vi "labview_python_send_serial_hex.vi"() -> ()   [LabVIEW 2025]
panel:
  in  "H2 Order":dbl
  in  "H2 Phase":dbl
  in  "H2 Volt":dbl
  in  "H1 Order":dbl
  in  "H1 Phase":dbl
  in  "H1 Volt":dbl
  in  "Freq Dev":dbl
  in  "Mod Freq":dbl
  in  "Mod Amp":dbl
  in  "ROCOF rate":dbl
  in  "Time":dbl
  in  "Frequency Step":dbl
  in  "Phase Step":dbl
  in  "Voltage Step":dbl
  in  "Test Type":u16(ring) items=["Steady State", "Voltage Step", "Phase Step", "Frequency Step", "Frequency Ramp", "Amplitude Modulation", "Phase Modulation", "Harmonics"]
  in  "Phase":dbl=90.0
  in  "Frequency":dbl=50.0
  in  "Voltage":dbl=1.0
  out "Debug":string
  in  "Python Version":T1(ring)=enum."3.12"
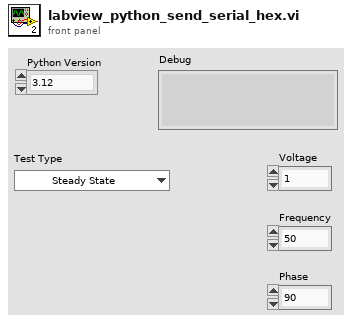
[diagram p1: front panel]
types:
  T1 = enum16{"3.6", "3.7", "3.8", "3.9", "3.10", "3.11", "3.12"}
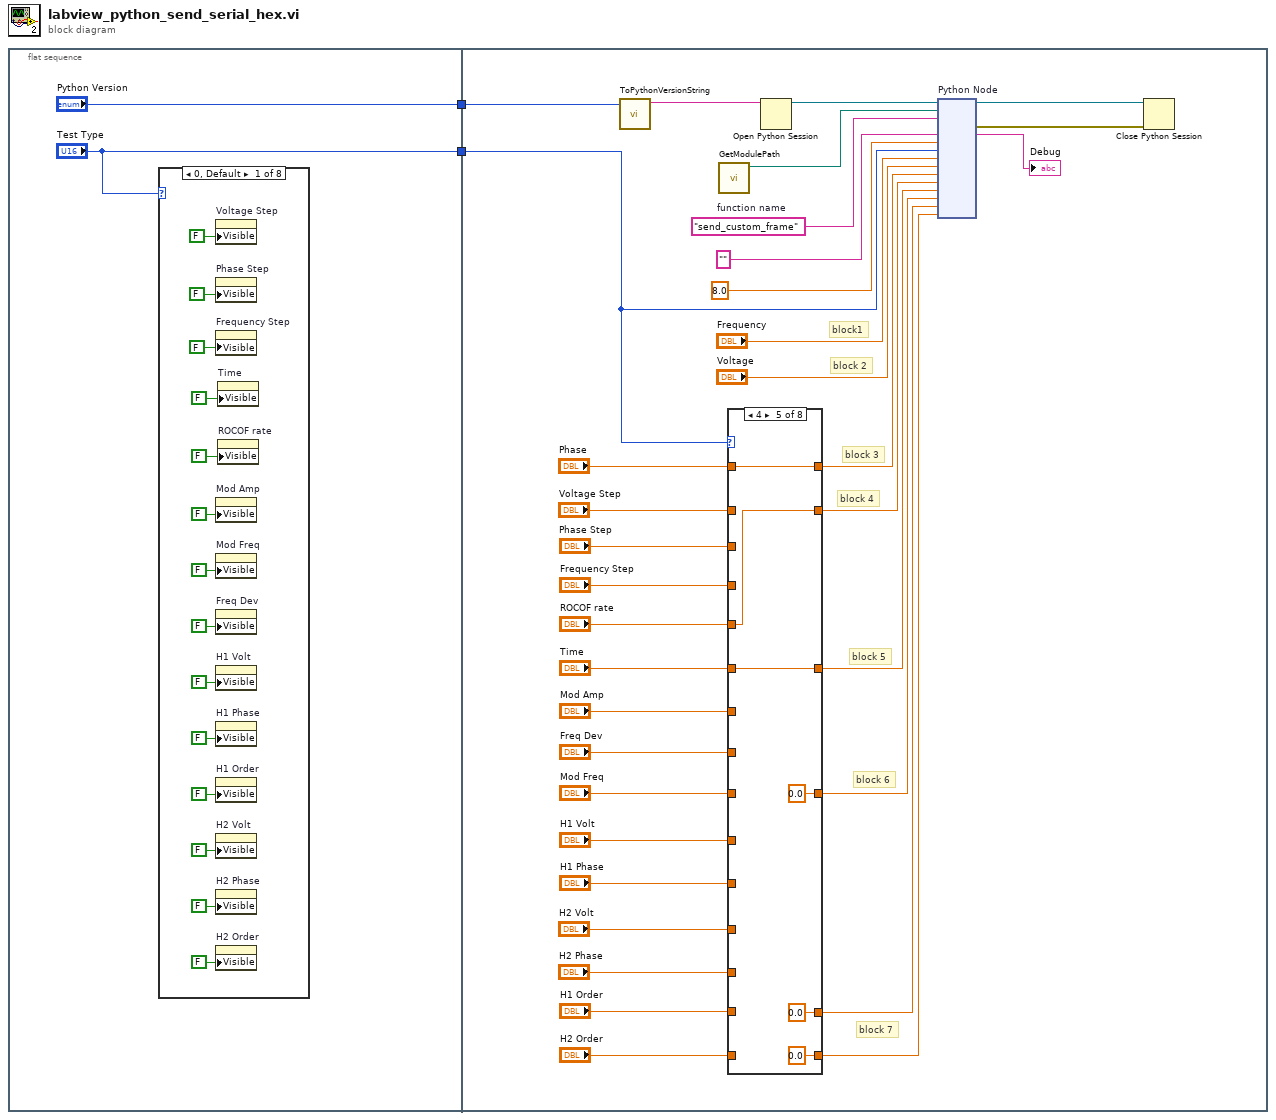
[diagram p0: block diagram]
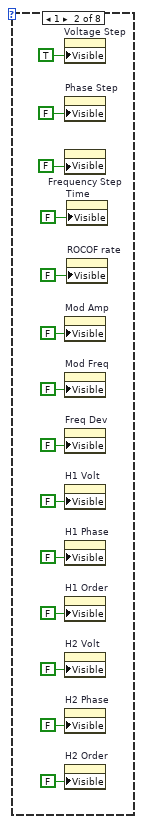
[diagram p2: hidden frame]
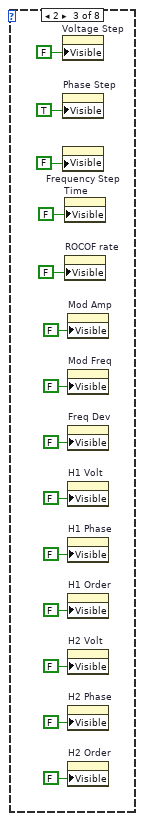
[diagram p3: hidden frame]
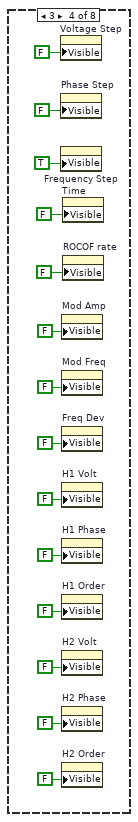
[diagram p4: hidden frame]
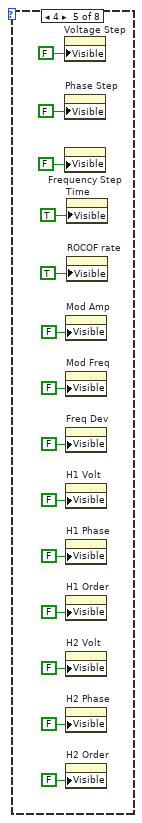
[diagram p5: hidden frame]
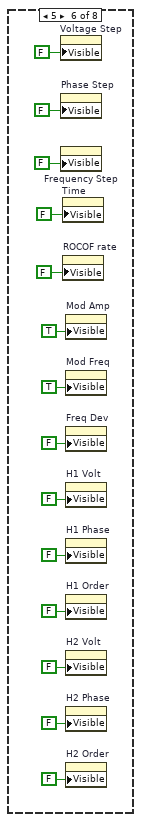
[diagram p6: hidden frame]
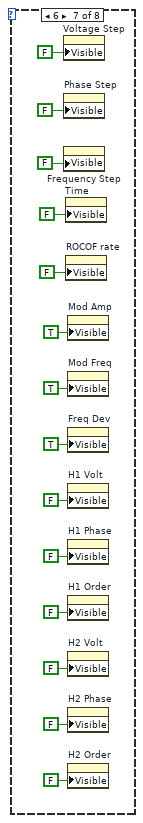
[diagram p7: hidden frame]
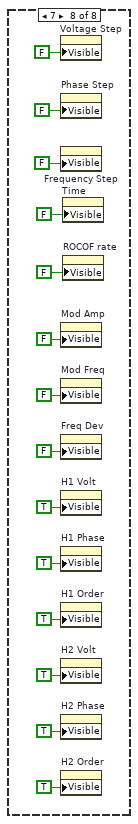
[diagram p8: hidden frame]
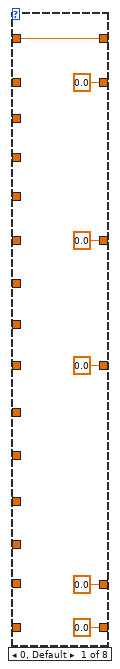
[diagram p9: hidden frame]
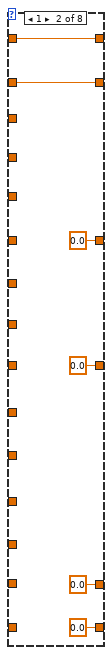
[diagram p10: hidden frame]
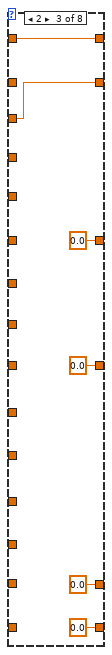
[diagram p11: hidden frame]
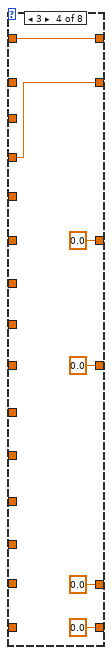
[diagram p12: hidden frame]
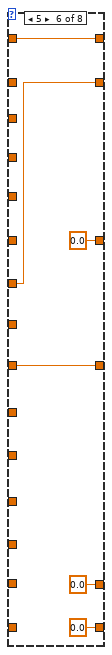
[diagram p13: hidden frame]
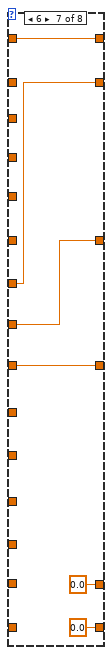
[diagram p14: hidden frame]
diagram:
  n1 = flat-sequence {
    tunnel: ["Python Version"] -> w2
    tunnel: ["Test Type"] -> w1
    tunnel: w2 -> [w142]
    tunnel: w1 -> [w138]
    frame #0 {
      n2 = case shown="0, Default" "Test Type" {
        frame 0, Default {
          n3 = property on="Voltage Step" class="DigNum (strict)"("Visible"=FALSE) -> ()  [unwired: 2 in, 2 out]
          n4 = property on="Phase Step" class="DigNum (strict)"("Visible"=FALSE) -> ()  [unwired: 2 in, 2 out]
          n5 = property on="Frequency Step" class="DigNum (strict)"("Visible"=FALSE) -> ()  [unwired: 2 in, 2 out]
          n6 = property on="Mod Amp" class="DigNum (strict)"("Visible"=FALSE) -> ()  [unwired: 2 in, 2 out]
          n7 = property on="Mod Freq" class="DigNum (strict)"("Visible"=FALSE) -> ()  [unwired: 2 in, 2 out]
          n8 = property on="Freq Dev" class="DigNum (strict)"("Visible"=FALSE) -> ()  [unwired: 2 in, 2 out]
          n9 = property on="H1 Volt" class="DigNum (strict)"("Visible"=FALSE) -> ()  [unwired: 2 in, 2 out]
          n10 = property on="H1 Phase" class="DigNum (strict)"("Visible"=FALSE) -> ()  [unwired: 2 in, 2 out]
          n11 = property on="H1 Order" class="DigNum (strict)"("Visible"=FALSE) -> ()  [unwired: 2 in, 2 out]
          n12 = property on="H2 Volt" class="DigNum (strict)"("Visible"=FALSE) -> ()  [unwired: 2 in, 2 out]
          n13 = property on="H2 Phase" class="DigNum (strict)"("Visible"=FALSE) -> ()  [unwired: 2 in, 2 out]
          n14 = property on="H2 Order" class="DigNum (strict)"("Visible"=FALSE) -> ()  [unwired: 2 in, 2 out]
          n15 = property on="Time" class="DigNum (strict)"("Visible"=FALSE) -> ()  [unwired: 2 in, 2 out]
          n16 = property on="ROCOF rate" class="DigNum (strict)"("Visible"=FALSE) -> ()  [unwired: 2 in, 2 out]
        }
        frame 1 {
          n17 = property on="Voltage Step" class="DigNum (strict)"("Visible"=TRUE) -> ()  [unwired: 2 in, 2 out]
          n18 = property on="Phase Step" class="DigNum (strict)"("Visible"=FALSE) -> ()  [unwired: 2 in, 2 out]
          n19 = property on="Frequency Step" class="DigNum (strict)"("Visible"=FALSE) -> ()  [unwired: 2 in, 2 out]
          n20 = property on="Mod Amp" class="DigNum (strict)"("Visible"=FALSE) -> ()  [unwired: 2 in, 2 out]
          n21 = property on="Mod Freq" class="DigNum (strict)"("Visible"=FALSE) -> ()  [unwired: 2 in, 2 out]
          n22 = property on="Freq Dev" class="DigNum (strict)"("Visible"=FALSE) -> ()  [unwired: 2 in, 2 out]
          n23 = property on="H1 Volt" class="DigNum (strict)"("Visible"=FALSE) -> ()  [unwired: 2 in, 2 out]
          n24 = property on="H1 Phase" class="DigNum (strict)"("Visible"=FALSE) -> ()  [unwired: 2 in, 2 out]
          n25 = property on="H1 Order" class="DigNum (strict)"("Visible"=FALSE) -> ()  [unwired: 2 in, 2 out]
          n26 = property on="H2 Volt" class="DigNum (strict)"("Visible"=FALSE) -> ()  [unwired: 2 in, 2 out]
          n27 = property on="H2 Phase" class="DigNum (strict)"("Visible"=FALSE) -> ()  [unwired: 2 in, 2 out]
          n28 = property on="H2 Order" class="DigNum (strict)"("Visible"=FALSE) -> ()  [unwired: 2 in, 2 out]
          n29 = property on="Time" class="DigNum (strict)"("Visible"=FALSE) -> ()  [unwired: 2 in, 2 out]
          n30 = property on="ROCOF rate" class="DigNum (strict)"("Visible"=FALSE) -> ()  [unwired: 2 in, 2 out]
        }
        frame 2 {
          n31 = property on="Voltage Step" class="DigNum (strict)"("Visible"=FALSE) -> ()  [unwired: 2 in, 2 out]
          n32 = property on="Phase Step" class="DigNum (strict)"("Visible"=TRUE) -> ()  [unwired: 2 in, 2 out]
          n33 = property on="Frequency Step" class="DigNum (strict)"("Visible"=FALSE) -> ()  [unwired: 2 in, 2 out]
          n34 = property on="Time" class="DigNum (strict)"("Visible"=FALSE) -> ()  [unwired: 2 in, 2 out]
          n35 = property on="ROCOF rate" class="DigNum (strict)"("Visible"=FALSE) -> ()  [unwired: 2 in, 2 out]
          n36 = property on="Mod Amp" class="DigNum (strict)"("Visible"=FALSE) -> ()  [unwired: 2 in, 2 out]
          n37 = property on="Mod Freq" class="DigNum (strict)"("Visible"=FALSE) -> ()  [unwired: 2 in, 2 out]
          n38 = property on="Freq Dev" class="DigNum (strict)"("Visible"=FALSE) -> ()  [unwired: 2 in, 2 out]
          n39 = property on="H1 Volt" class="DigNum (strict)"("Visible"=FALSE) -> ()  [unwired: 2 in, 2 out]
          n40 = property on="H1 Phase" class="DigNum (strict)"("Visible"=FALSE) -> ()  [unwired: 2 in, 2 out]
          n41 = property on="H1 Order" class="DigNum (strict)"("Visible"=FALSE) -> ()  [unwired: 2 in, 2 out]
          n42 = property on="H2 Volt" class="DigNum (strict)"("Visible"=FALSE) -> ()  [unwired: 2 in, 2 out]
          n43 = property on="H2 Phase" class="DigNum (strict)"("Visible"=FALSE) -> ()  [unwired: 2 in, 2 out]
          n44 = property on="H2 Order" class="DigNum (strict)"("Visible"=FALSE) -> ()  [unwired: 2 in, 2 out]
        }
        frame 3 {
          n45 = property on="Voltage Step" class="DigNum (strict)"("Visible"=FALSE) -> ()  [unwired: 2 in, 2 out]
          n46 = property on="Phase Step" class="DigNum (strict)"("Visible"=FALSE) -> ()  [unwired: 2 in, 2 out]
          n47 = property on="Frequency Step" class="DigNum (strict)"("Visible"=TRUE) -> ()  [unwired: 2 in, 2 out]
          n48 = property on="Mod Amp" class="DigNum (strict)"("Visible"=FALSE) -> ()  [unwired: 2 in, 2 out]
          n49 = property on="Mod Freq" class="DigNum (strict)"("Visible"=FALSE) -> ()  [unwired: 2 in, 2 out]
          n50 = property on="Freq Dev" class="DigNum (strict)"("Visible"=FALSE) -> ()  [unwired: 2 in, 2 out]
          n51 = property on="H1 Volt" class="DigNum (strict)"("Visible"=FALSE) -> ()  [unwired: 2 in, 2 out]
          n52 = property on="H1 Phase" class="DigNum (strict)"("Visible"=FALSE) -> ()  [unwired: 2 in, 2 out]
          n53 = property on="H1 Order" class="DigNum (strict)"("Visible"=FALSE) -> ()  [unwired: 2 in, 2 out]
          n54 = property on="H2 Volt" class="DigNum (strict)"("Visible"=FALSE) -> ()  [unwired: 2 in, 2 out]
          n55 = property on="H2 Phase" class="DigNum (strict)"("Visible"=FALSE) -> ()  [unwired: 2 in, 2 out]
          n56 = property on="H2 Order" class="DigNum (strict)"("Visible"=FALSE) -> ()  [unwired: 2 in, 2 out]
          n57 = property on="Time" class="DigNum (strict)"("Visible"=FALSE) -> ()  [unwired: 2 in, 2 out]
          n58 = property on="ROCOF rate" class="DigNum (strict)"("Visible"=FALSE) -> ()  [unwired: 2 in, 2 out]
        }
        frame 4 {
          n59 = property on="Voltage Step" class="DigNum (strict)"("Visible"=FALSE) -> ()  [unwired: 2 in, 2 out]
          n60 = property on="Phase Step" class="DigNum (strict)"("Visible"=FALSE) -> ()  [unwired: 2 in, 2 out]
          n61 = property on="Frequency Step" class="DigNum (strict)"("Visible"=FALSE) -> ()  [unwired: 2 in, 2 out]
          n62 = property on="Mod Amp" class="DigNum (strict)"("Visible"=FALSE) -> ()  [unwired: 2 in, 2 out]
          n63 = property on="Mod Freq" class="DigNum (strict)"("Visible"=FALSE) -> ()  [unwired: 2 in, 2 out]
          n64 = property on="Freq Dev" class="DigNum (strict)"("Visible"=FALSE) -> ()  [unwired: 2 in, 2 out]
          n65 = property on="H1 Volt" class="DigNum (strict)"("Visible"=FALSE) -> ()  [unwired: 2 in, 2 out]
          n66 = property on="H1 Phase" class="DigNum (strict)"("Visible"=FALSE) -> ()  [unwired: 2 in, 2 out]
          n67 = property on="H1 Order" class="DigNum (strict)"("Visible"=FALSE) -> ()  [unwired: 2 in, 2 out]
          n68 = property on="H2 Volt" class="DigNum (strict)"("Visible"=FALSE) -> ()  [unwired: 2 in, 2 out]
          n69 = property on="H2 Phase" class="DigNum (strict)"("Visible"=FALSE) -> ()  [unwired: 2 in, 2 out]
          n70 = property on="H2 Order" class="DigNum (strict)"("Visible"=FALSE) -> ()  [unwired: 2 in, 2 out]
          n71 = property on="Time" class="DigNum (strict)"("Visible"=TRUE) -> ()  [unwired: 2 in, 2 out]
          n72 = property on="ROCOF rate" class="DigNum (strict)"("Visible"=TRUE) -> ()  [unwired: 2 in, 2 out]
        }
        frame 5 {
          n73 = property on="Voltage Step" class="DigNum (strict)"("Visible"=FALSE) -> ()  [unwired: 2 in, 2 out]
          n74 = property on="Phase Step" class="DigNum (strict)"("Visible"=FALSE) -> ()  [unwired: 2 in, 2 out]
          n75 = property on="Frequency Step" class="DigNum (strict)"("Visible"=FALSE) -> ()  [unwired: 2 in, 2 out]
          n76 = property on="Time" class="DigNum (strict)"("Visible"=FALSE) -> ()  [unwired: 2 in, 2 out]
          n77 = property on="ROCOF rate" class="DigNum (strict)"("Visible"=FALSE) -> ()  [unwired: 2 in, 2 out]
          n78 = property on="Mod Amp" class="DigNum (strict)"("Visible"=TRUE) -> ()  [unwired: 2 in, 2 out]
          n79 = property on="Mod Freq" class="DigNum (strict)"("Visible"=TRUE) -> ()  [unwired: 2 in, 2 out]
          n80 = property on="Freq Dev" class="DigNum (strict)"("Visible"=FALSE) -> ()  [unwired: 2 in, 2 out]
          n81 = property on="H1 Volt" class="DigNum (strict)"("Visible"=FALSE) -> ()  [unwired: 2 in, 2 out]
          n82 = property on="H1 Phase" class="DigNum (strict)"("Visible"=FALSE) -> ()  [unwired: 2 in, 2 out]
          n83 = property on="H1 Order" class="DigNum (strict)"("Visible"=FALSE) -> ()  [unwired: 2 in, 2 out]
          n84 = property on="H2 Volt" class="DigNum (strict)"("Visible"=FALSE) -> ()  [unwired: 2 in, 2 out]
          n85 = property on="H2 Phase" class="DigNum (strict)"("Visible"=FALSE) -> ()  [unwired: 2 in, 2 out]
          n86 = property on="H2 Order" class="DigNum (strict)"("Visible"=FALSE) -> ()  [unwired: 2 in, 2 out]
        }
        frame 6 {
          n87 = property on="Voltage Step" class="DigNum (strict)"("Visible"=FALSE) -> ()  [unwired: 2 in, 2 out]
          n88 = property on="Phase Step" class="DigNum (strict)"("Visible"=FALSE) -> ()  [unwired: 2 in, 2 out]
          n89 = property on="Frequency Step" class="DigNum (strict)"("Visible"=FALSE) -> ()  [unwired: 2 in, 2 out]
          n90 = property on="Time" class="DigNum (strict)"("Visible"=FALSE) -> ()  [unwired: 2 in, 2 out]
          n91 = property on="ROCOF rate" class="DigNum (strict)"("Visible"=FALSE) -> ()  [unwired: 2 in, 2 out]
          n92 = property on="Mod Amp" class="DigNum (strict)"("Visible"=TRUE) -> ()  [unwired: 2 in, 2 out]
          n93 = property on="Mod Freq" class="DigNum (strict)"("Visible"=TRUE) -> ()  [unwired: 2 in, 2 out]
          n94 = property on="Freq Dev" class="DigNum (strict)"("Visible"=TRUE) -> ()  [unwired: 2 in, 2 out]
          n95 = property on="H1 Volt" class="DigNum (strict)"("Visible"=FALSE) -> ()  [unwired: 2 in, 2 out]
          n96 = property on="H1 Phase" class="DigNum (strict)"("Visible"=FALSE) -> ()  [unwired: 2 in, 2 out]
          n97 = property on="H1 Order" class="DigNum (strict)"("Visible"=FALSE) -> ()  [unwired: 2 in, 2 out]
          n98 = property on="H2 Volt" class="DigNum (strict)"("Visible"=FALSE) -> ()  [unwired: 2 in, 2 out]
          n99 = property on="H2 Phase" class="DigNum (strict)"("Visible"=FALSE) -> ()  [unwired: 2 in, 2 out]
          n100 = property on="H2 Order" class="DigNum (strict)"("Visible"=FALSE) -> ()  [unwired: 2 in, 2 out]
        }
        frame 7 {
          n101 = property on="Voltage Step" class="DigNum (strict)"("Visible"=FALSE) -> ()  [unwired: 2 in, 2 out]
          n102 = property on="Phase Step" class="DigNum (strict)"("Visible"=FALSE) -> ()  [unwired: 2 in, 2 out]
          n103 = property on="Frequency Step" class="DigNum (strict)"("Visible"=FALSE) -> ()  [unwired: 2 in, 2 out]
          n104 = property on="Mod Amp" class="DigNum (strict)"("Visible"=FALSE) -> ()  [unwired: 2 in, 2 out]
          n105 = property on="Mod Freq" class="DigNum (strict)"("Visible"=FALSE) -> ()  [unwired: 2 in, 2 out]
          n106 = property on="Freq Dev" class="DigNum (strict)"("Visible"=FALSE) -> ()  [unwired: 2 in, 2 out]
          n107 = property on="H1 Volt" class="DigNum (strict)"("Visible"=TRUE) -> ()  [unwired: 2 in, 2 out]
          n108 = property on="H1 Phase" class="DigNum (strict)"("Visible"=TRUE) -> ()  [unwired: 2 in, 2 out]
          n109 = property on="H1 Order" class="DigNum (strict)"("Visible"=TRUE) -> ()  [unwired: 2 in, 2 out]
          n110 = property on="H2 Volt" class="DigNum (strict)"("Visible"=TRUE) -> ()  [unwired: 2 in, 2 out]
          n111 = property on="H2 Phase" class="DigNum (strict)"("Visible"=TRUE) -> ()  [unwired: 2 in, 2 out]
          n112 = property on="H2 Order" class="DigNum (strict)"("Visible"=TRUE) -> ()  [unwired: 2 in, 2 out]
          n113 = property on="Time" class="DigNum (strict)"("Visible"=FALSE) -> ()  [unwired: 2 in, 2 out]
          n114 = property on="ROCOF rate" class="DigNum (strict)"("Visible"=FALSE) -> ()  [unwired: 2 in, 2 out]
        }
      }
    }
    frame #1 {
      w144 = "send_custom_frame"  # function name
      # "block 7"
      # "block 6"
      # "block 5"
      # "block 4"
      # "block 3"
      # "block 2"
      # "block1"
      n115 = call "ToPythonVersionString.vi"("python version"=w142) -> ("python version string"=w150:string)  [unwired: 10 in]
      n116 = call "GetModulePath.vi"() -> ("module path"=w149:path)  [unwired: 11 in]
      n117 = case shown="4" w138 {
        tunnel: "Voltage Step" -> [_ w162 _ _ _ _ _ _]
        tunnel: "Phase Step" -> [_ _ w168 _ _ _ _ _]
        tunnel: "Frequency Step" -> [_ _ _ w174 _ _ _ _]
        tunnel: "ROCOF rate" -> [_ _ _ _ w180 _ _ _]
        tunnel: [0.0 ("ROCOF rate") w162 w168 w174 w180 w184 w191 w195] -> w133
        tunnel: "Time" -> [_ _ _ _ w179 _ _ _]
        tunnel: [0.0 ("Time") 0.0 ("Time") 0.0 ("Time") 0.0 ("Time") w179 0.0 ("Time") w189 w196] -> w131
        tunnel: "Mod Amp" -> [_ _ _ _ _ w184 w191 _]
        tunnel: "Mod Freq" -> [_ _ _ _ _ w185 w190 _]
        tunnel: "H1 Volt" -> [_ _ _ _ _ _ _ w194]
        tunnel: "H1 Phase" -> [_ _ _ _ _ _ _ w195]
        tunnel: "H2 Volt" -> [_ _ _ _ _ _ _ w196]
        tunnel: "H2 Phase" -> [_ _ _ _ _ _ _ w197]
        tunnel: "H2 Order" -> [_ _ _ _ _ _ _ w198]
        tunnel: "Phase" -> [w154 w160 w166 w172 w178 w186 w192 _]
        tunnel: [w154 w160 w166 w172 w178 w186 w192 w194] -> w122
        tunnel: [0.0 ("H2 Phase") 0.0 ("H2 Phase") 0.0 ("H2 Phase") 0.0 ("H2 Phase") 0.0 ("H2 Phase") w185 w190 w197] -> w121
        tunnel: "Freq Dev" -> [_ _ _ _ _ _ w189 _]
        tunnel: [0.0 ("H2 Order") 0.0 ("H2 Order") 0.0 ("H2 Order") 0.0 ("H2 Order") 0.0 ("H2 Order") 0.0 ("H2 Order") 0.0 ("H2 Order") w198] -> w117
        tunnel: "H1 Order" -> [_ _ _ _ _ _ _ w193]
        tunnel: [0.0 ("H1 Order") 0.0 ("H1 Order") 0.0 ("H1 Order") 0.0 ("H1 Order") 0.0 ("H1 Order") 0.0 ("H1 Order") 0.0 ("H1 Order") w193] -> w118
        frame 0, Default {
        }
        frame 1 {
        }
        frame 2 {
        }
        frame 3 {
        }
        frame 4 {
        }
        frame 5 {
        }
        frame 6 {
        }
        frame 7 {
        }
      }
      n118 = Open Python Session(python version=w150) -> (session out=w146:refnum<k35>)  [unwired: 2 in, 1 out]
      n119 = node "Python Node"(w146, w149, w144, "", 8.0, w138, "Frequency", "Voltage", w122, w133, w131, w121, w118, w117) -> (w147:refnum<k35>, w148:errorcluster, →"Debug":string)  [unwired: 11 in, 2 out]
      n120 = Close Python Session(session in=w147, error in=w148) -> ()  [unwired: 1 out]
    }
  }
